vi "ProdaNG.TestStepResult.Set.vi"(8 "error in (no error)":errorcluster, 9 "isRepeat (0)":i32, 10 "TestStepResult":T1, 11 "dbHandle":i32) -> (0 "error out":errorcluster, 3 "dbHandle":i32)   [LabVIEW 2016]
doc: "This function changes the process step result, which is defined by a ProcessStepResult structure. A process step result can either be set intentionally or leave the check of the test step results and the resulting changes to the DLL. In case, that the DLL changes the Process Result, the mdTime of the according Product is set to the current time and the mdProcessStepId is set to this process step. \nThe automatic check stands to the following rule:\n1. It is checked, if all test steps have the Status IO.\nIf the result of the test is IO, the status 1 (IO) is set in the test value result, otherwise the status 0 (NIO), respective 5 (IO Repeat) or 6 (NIO Repeat) in case of a repeat.\nParameter:\nhandle is an Integer, which is returned by the function Login() at the creation of a new connection.\nisRepeat shows, if this step is a repeat.\nprocessStepResult is a pointer on a ProcessStepResult structure, which elements must be prefilled. The structure must be defined and filled in the calling program. Changes can only be made on the elements StatusId, startTime and endTime. If the Endtime is not set, it is automatically filled with the current time by the DLL. \nThe element statusId is of particular importance:\nIf this element is passed with the value -1, the DLL makes a check on the test step results and sets the changeable elements automatically. Otherwise the returned values for status, start time and end time are set.\n\nReturncodes:\n0 No error\n< 0 ORACLE Error code\n6 (ERROR_INVALID_HANDLE) in case of an invalid handle\n1403 Record does not exist"
uses:
  Controls/ProdaNG.TestStepResult.ctl
  Controls/ProdaNG.TestStepResultSize.ctl
  prodllNG.dll
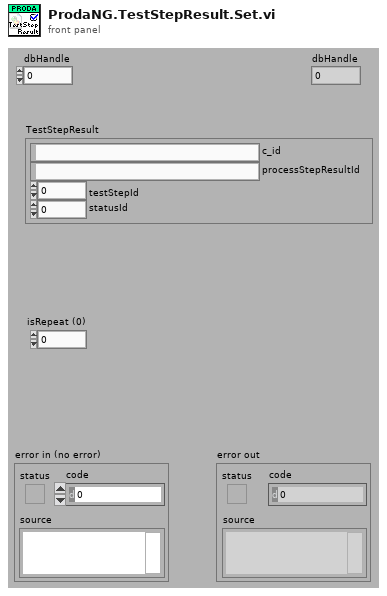
[diagram p1: front panel]
types:
  T1 = typedef "ProdaNG.TestStepResult.ctl" = cluster{"c_id":string, "processStepResultId":string, "testStepId":i32, "statusId":i32}
  T2 = typedef "ProdaNG.TestStepResultSize.ctl" = cluster{"c_id":i32, "processStepResultId":i32, "testStepId":i32, "statusId":i32}
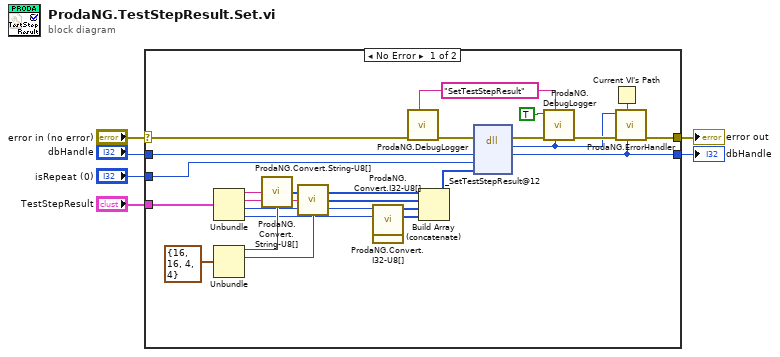
[diagram p0: block diagram]
diagram:
  n1 = case shown="No Error" "error in (no error)" {
    selector: "error in (no error)" -> [w13 w33]
    tunnel: [w9 w33] -> w5
    tunnel: [w8 w32] -> w4
    tunnel: "dbHandle" -> [w12 w32]
    tunnel: "isRepeat (0)" -> [w11 _]
    tunnel: "TestStepResult" -> [w10 _]
    frame No Error {
      w28 = "SetTestStepResult" ("cmd")
      n2 = Unbundle(w10) -> ("c_id"=w30:string, "processStepResultId"=w31:string, "testStepId"=w18:i32, "statusId"=w17:i32)
      n3 = Unbundle(T2 {"c_id"=16, "processStepResultId"=16, "testStepId"=4, "statusId"=4} ("TestStepResultSize")) -> ("c_id"=w22:i32, "processStepResultId"=w20:i32)  [unwired: 2 out]
      n4 = call "ProdaNG.Convert.String-U8[].vi"("Input String"=w30, "Size"=w22) -> ("Output"=w21:u8[])
      n5 = call "ProdaNG.Convert.String-U8[].vi"("Input String"=w31, "Size"=w20) -> ("Output"=w19:u8[])
      n6 = call "ProdaNG.Convert.I32-U8[].vi"("32bit integer"=w18) -> ("unsigned byte array"=w16:u8[])  [unwired: 10 in]
      n7 = call "ProdaNG.Convert.I32-U8[].vi"("32bit integer"=w17) -> ("unsigned byte array"=w15:u8[])  [unwired: 10 in]
      n8 = call "ProdaNG.DebugLogger.vi"("cmd"=w28, "error in (no error)"=w13) -> ("error out"=w23:errorcluster)  [unwired: 9 in]
      n9 = Build Array (concatenate)(w21, w19, w16, w15) -> (w14:u8[])
      n10 = dll-call lib="D:/svn/LineTraceSystem/SOFTWARE/sources/Database/ProdaNG/prodllNG.dll" fn="_SetTestStepResult@12" ("ProDll.dll:InitProDll")(error in=w23, "dbHandle"=w12, "isRepeat"=w11, "testStepResult"=w14) -> (error out=w26:errorcluster, "return type"=w24:i32, "dbHandle"=w8:i32)  [unwired: 4 in, 1 out]
      n11 = call "ProdaNG.DebugLogger.vi"("return type"=w24, "cmd"=w28, "error in (no error)"=w26, "done? (F)"=TRUE) -> ("error out"=w25:errorcluster)  [unwired: 7 in]
      n12 = Current VI's Path() -> (path=w29:path)
      n13 = call "ProdaNG.ErrorHandler.vi"("dbHandleIn"=w8, "Path"=w29, "error in"=w25, "output_parameter"=w24) -> ("error out"=w9:errorcluster)  [unwired: 7 in]
    }
    frame Error {
    }
  }
  "error out" <- w5
  "dbHandle" <- w4
